vi "BotSpeak_PWM.vi"(0 "Strength (100)":sgl=100.0, 2 "Bot Settings":T1, 3 "PWM Line":u8=3) -> (4 "Bot Settings out":T1)   [LabVIEW 2012]
doc: "Uses pulse width modulation to vary the voltage sent out the specified \"DIO Line\". \"Strength\" ranges from 0 to 100, and is a precentage of the max voltage that can be sent through the specified line."
uses:
  <userlib>/botspeak/VIs/Direct/BotSpeak_Control.ctl
panel:
  out "response":string
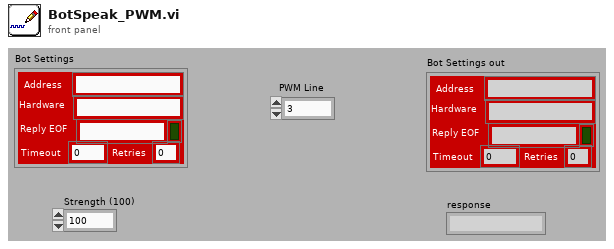
[diagram p1: front panel]
types:
  T1 = typedef "BotSpeak_Control.ctl" = cluster{"Address":string, "Reply EOF":string, "Hardware":string, "Retries":i8, "Timeout":i32, "Open?":bool}
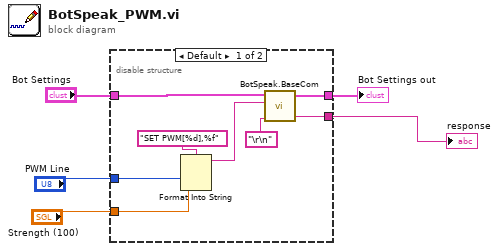
[diagram p0: block diagram]
diagram:
  n1 = disable-structure shown="Default" {
    disable-tunnel: "Bot Settings" -> [w10 _]
    disable-tunnel: [w9 _] -> w4
    disable-tunnel: [w8 _] -> w3
    disable-tunnel: "PWM Line" -> [w7 _]
    disable-tunnel: "Strength (100)" -> [w6 _]
    frame condition #0 (active) {
      n2 = Format Into String(format string="SET PWM[%d],%f" ("command"), w7, w6) -> (resulting string=w13:string)  [unwired: 2 in, 1 out]
      n3 = call <userlib>:"BotSpeak.BaseCom.vi"("Termination"="\r\n", "command"=w13, "Bot Settings in"=w10) -> ("response"=w8:string, "Bot Settings out"=w9:T1)  [unwired: 2 in]
    }
    frame condition #1 {
    }
  }
  "Bot Settings out" <- w4
  "response" <- w3
